vi "Get Primary Key.vi"(8 "error in (no error)":errorcluster, 10 "Table Name Array":string[](array[string]), 11 "Database Schema in":refnum<class "Database Adv Schema.lvclass">) -> (0 "error out":errorcluster, 1 "PK Found?":bool[](array[boolean]), 2 "Primary Key Array":T1[](array[typedef]), 3 "Database Schema out":refnum<class "Database Adv Schema.lvclass">)   [LabVIEW 2020, in "Database Interfaces.lvlib" / "Database Adv Schema.lvclass"]
uses:
  Database Adv Schema.lvclass
  Primary Key Info.ctl
  Database Interfaces.lvlib
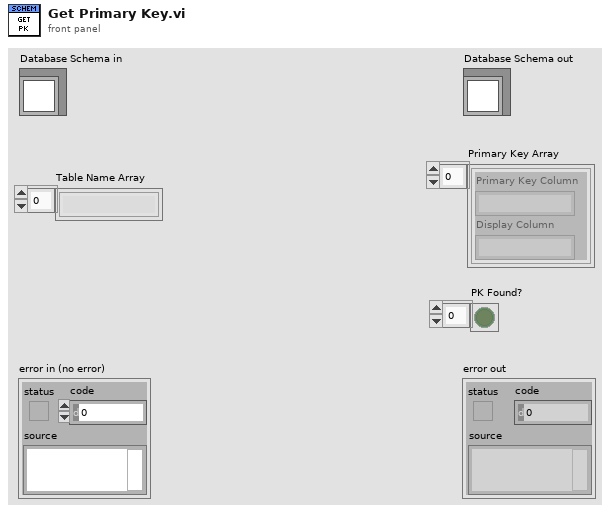
[diagram p1: front panel]
types:
  T1 = typedef "Database Interfaces.lvlib/Primary Key Info.ctl" = cluster{"Primary Key Column":string, "Display Column":string}
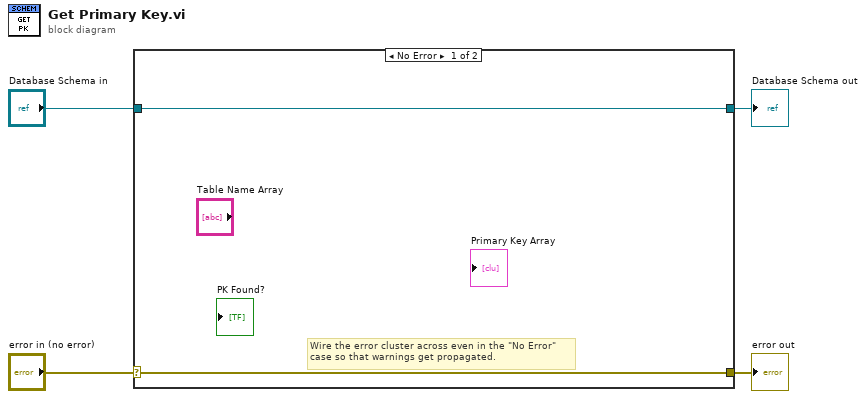
[diagram p0: block diagram]
diagram:
  n1 = case shown="No Error" "error in (no error)" {
    selector: "error in (no error)" -> [w5 w8]
    tunnel: [w5 w8] -> w3
    tunnel: [w6 w7] -> w1
    tunnel: "Database Schema in" -> [w6 w7]
    frame No Error {
      # "Wire the error cluster across even in the \"No Error\"\ncase so that warnings get propagated."
    }
    frame Error {
    }
  }
  "error out" <- w3
  "Database Schema out" <- w1
